vi "Convert_Version_ERD.vi"(0 "ERD Data Out":T1[](array[typedef]) {"ERD Number" format="%.0x"}, 11 "Error In":errorcluster) -> (4 "Version":T2, 15 "Error Out":errorcluster)   [LabVIEW 2016]
uses:
  type defs/Version.ctl
  Common/LabVIEW GEA2 Toolkit/LabVIEW_GEA2_Toolkit.lvlibp/type defs/ERD Read Data Out.ctl
  Common/LabVIEW GEA2 Toolkit/LabVIEW_GEA2_Toolkit.lvlibp
panel:
  # "Software Version"
  # "UI"
  # "MC"
  # "INV"
  # "PERSONALITY"
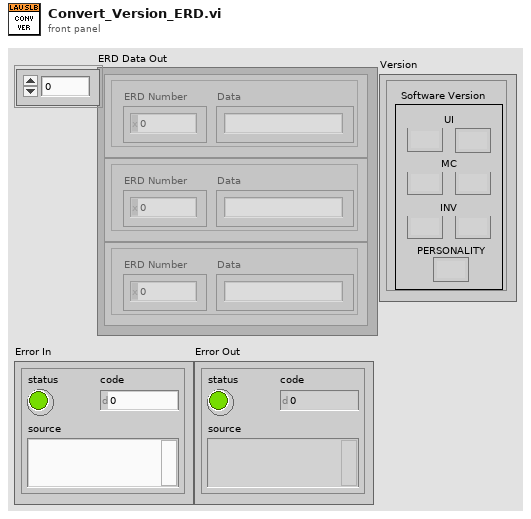
[diagram p1: front panel]
types:
  T1 = typedef "LabVIEW_GEA2_Toolkit.lvlibp/ERD Read Data Out.ctl" = cluster{"ERD Number":u16, "Data":string}
  T2 = typedef "Version.ctl" = cluster{"UI Major":string, "UI Minor":string, "MC Minor":string, "MC Major":string, "Inverter Minor":string, "Inverter Major":string, "Personality":string}
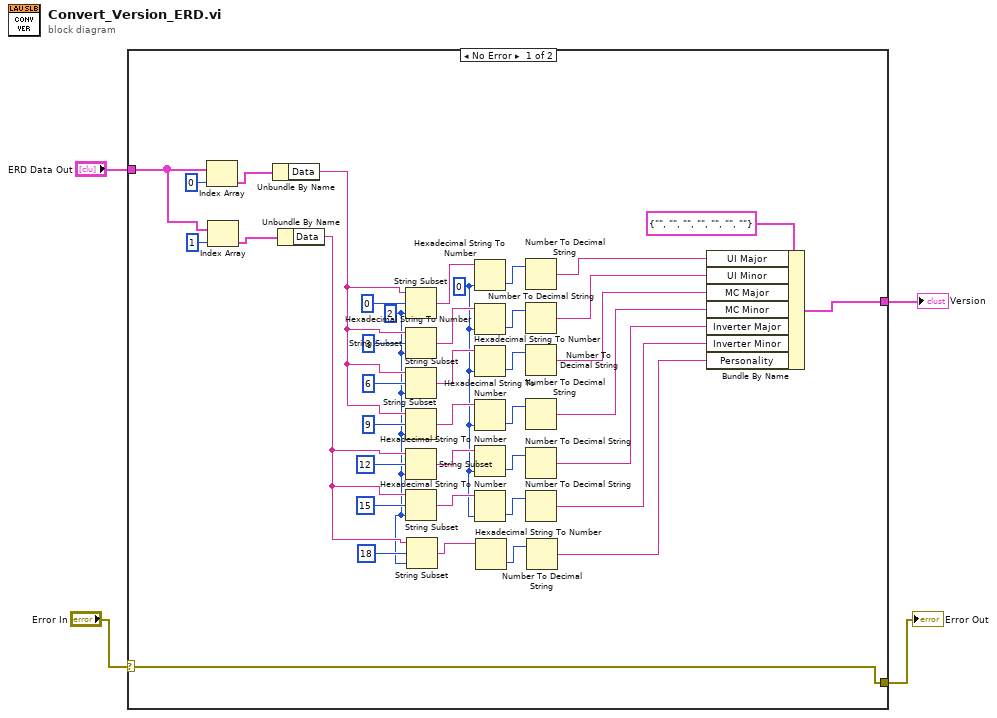
[diagram p0: block diagram]
diagram:
  n1 = case shown="No Error" "Error In" {
    selector: "Error In" -> [w13 w45]
    tunnel: [w13 w45] -> w3
    tunnel: [w23 _] -> w2
    tunnel: "ERD Data Out" -> [w18 _]
    frame No Error {
      w12 = u8 0 ("length (rest)")
      w5 = 2 ("length (rest)")
      n2 = Index Array(array=w18, index=0) -> (element=w17:T1)
      n3 = Index Array(array=w18, index=1) -> (element=w16:T1)
      n4 = Unbundle By Name(w17) -> ("Data"=w14:string)
      n5 = Unbundle By Name(w16) -> ("Data"=w6:string)
      n6 = String Subset(string=w14, offset (0)=0 ("length (rest)"), length (rest)=w5) -> (substring=w43:string)
      n7 = String Subset(string=w14, offset (0)=3 ("length (rest)"), length (rest)=w5) -> (substring=w37:string)
      n8 = String Subset(string=w14, offset (0)=6 ("length (rest)"), length (rest)=w5) -> (substring=w22:string)
      n9 = String Subset(string=w14, offset (0)=9 ("length (rest)"), length (rest)=w5) -> (substring=w21:string)
      n10 = String Subset(string=w6, offset (0)=12 ("length (rest)"), length (rest)=w5) -> (substring=w36:string)
      n11 = String Subset(string=w6, offset (0)=15 ("length (rest)"), length (rest)=w5) -> (substring=w35:string)
      n12 = String Subset(string=w6, offset (0)=18 ("length (rest)"), length (rest)=w5) -> (substring=w9:string)
      n13 = Hexadecimal String To Number(string=w43, default (0uL)=w12) -> (number=w34:u8)  [unwired: 1 in, 1 out]
      n14 = Hexadecimal String To Number(string=w37, default (0uL)=w12) -> (number=w33:u8)  [unwired: 1 in, 1 out]
      n15 = Hexadecimal String To Number(string=w22, default (0uL)=w12) -> (number=w32:u8)  [unwired: 1 in, 1 out]
      n16 = Hexadecimal String To Number(string=w21, default (0uL)=w12) -> (number=w31:u8)  [unwired: 1 in, 1 out]
      n17 = Hexadecimal String To Number(string=w36, default (0uL)=w12) -> (number=w30:u8)  [unwired: 1 in, 1 out]
      n18 = Hexadecimal String To Number(string=w35, default (0uL)=w12) -> (number=w10:u8)  [unwired: 1 in, 1 out]
      n19 = Hexadecimal String To Number(string=w9) -> (number=w8:u32)  [unwired: 2 in, 1 out]
      n20 = Number To Decimal String(number=w34) -> (decimal integer string=w24:string)  [unwired: 1 in]
      n21 = Number To Decimal String(number=w33) -> (decimal integer string=w25:string)  [unwired: 1 in]
      n22 = Number To Decimal String(number=w32) -> (decimal integer string=w26:string)  [unwired: 1 in]
      n23 = Number To Decimal String(number=w31) -> (decimal integer string=w27:string)  [unwired: 1 in]
      n24 = Number To Decimal String(number=w30) -> (decimal integer string=w28:string)  [unwired: 1 in]
      n25 = Number To Decimal String(number=w10) -> (decimal integer string=w29:string)  [unwired: 1 in]
      n26 = Number To Decimal String(number=w8) -> (decimal integer string=w7:string)  [unwired: 1 in]
      n27 = Bundle By Name(cluster=T2 {"UI Major"="", "UI Minor"="", "MC Minor"="", "MC Major"="", "Inverter Minor"="", "Inverter Major"="", "Personality"=""} ("Version"), "UI Major"=w24, "UI Minor"=w25, "MC Major"=w26, "MC Minor"=w27, "Inverter Major"=w28, "Inverter Minor"=w29, "Personality"=w7) -> (w23:T2)
    }
    frame Error {
    }
  }
  "Error Out" <- w3
  "Version" <- w2
